vi "Write Qex.vi"(8 "error in (no error)":errorcluster, 10 "Qex":dbl, 11 "DMA in":refnum<class "DMA.lvclass">) -> (0 "error out":errorcluster, 3 "DMA out":refnum<class "DMA.lvclass">)   [LabVIEW 2014, in "DMA.lvclass"]
uses:
  DMA.lvclass
  DMA.lvclass/DMA.ctl
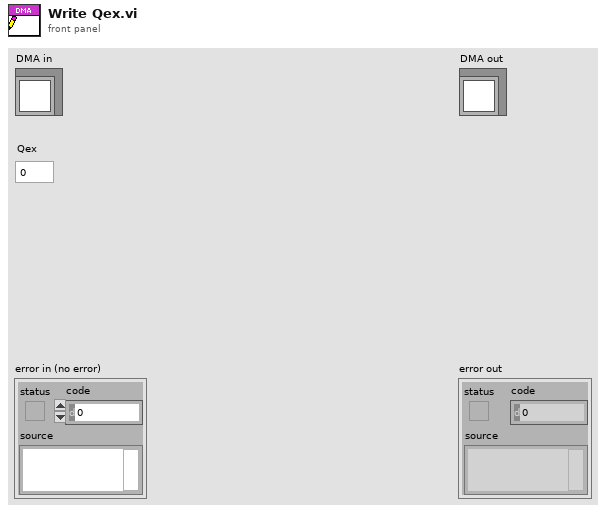
[diagram p1: front panel]
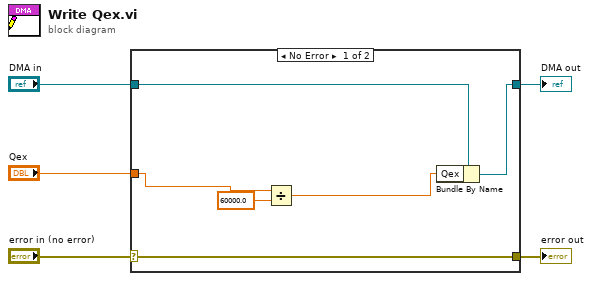
[diagram p0: block diagram]
diagram:
  n1 = case shown="No Error" "error in (no error)" {
    selector: "error in (no error)" -> [w11 w12]
    tunnel: [w11 w12] -> w4
    tunnel: [w9 w13] -> w2
    tunnel: "DMA in" -> [w10 w13]
    tunnel: "Qex" -> [w7 _]
    frame No Error {
      n2 = Divide(x=w7, y=60000.0) -> (x/y=w6:dbl)
      n3 = Bundle By Name(cluster=w10, "Qex"=w6) -> (w9:refnum<class "DMA.lvclass">)
    }
    frame Error {
    }
  }
  "error out" <- w4
  "DMA out" <- w2
